vi "emi_ Loop multi error state monitor.vi"(5 "Loop ID in":u16, 9 "error in (no error)":errorcluster, 12 "Loc Sub ID":u16, 13 "Elevated priority":bool) -> (6 "Loop ID out":u16, 10 "error out":errorcluster)   [LabVIEW 2011]
doc: "Monitors severl error states based on sub id. Sends a message when any of them changes.\n\nDoes not remove teh errors"
uses:
  emi_Read System ID.vi
  Private/_emi_GFV System ID.vi
  <vilib>/Utility/error.llb/Clear Errors.vi
  S&E reporting/Private/_emi_S&E Q Generator.vi
panel:
  # "Always uses Sub ID 0."
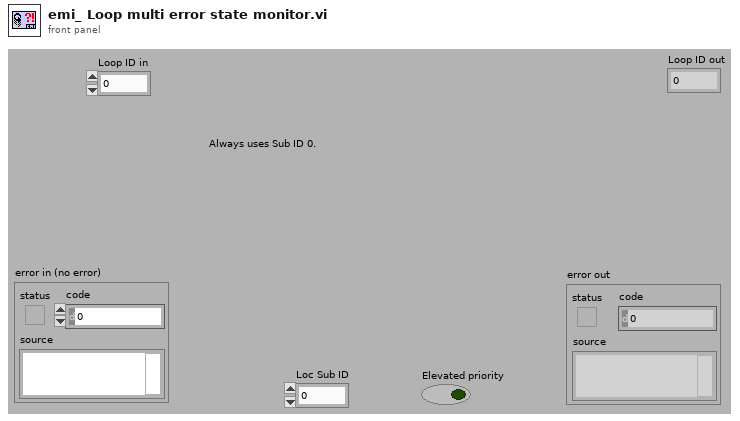
[diagram p1: front panel]
types:
  T1 = cluster{"error in (no error)":errorcluster, "Elevated priority":bool}
  T2 = cluster{"error in (no error)":errorcluster, "Elevated priority":bool}[]
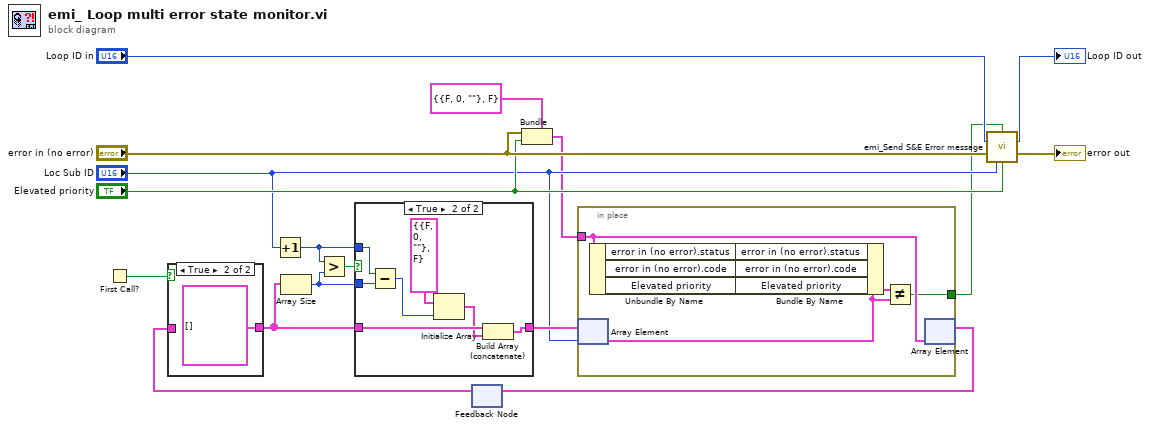
[diagram p0: block diagram]
diagram:
  n1 = First Call?() -> (First Call?: T/F=w8:bool)
  n2 = Increment(x="Loc Sub ID") -> (x+1=w9:u16)
  n3 = feedback #1() -> (w7:T2)  [unwired: 1 in]
  n4 = case shown="True" w8 {
    tunnel: [w18 T2 []] -> w6
    tunnel: w7 -> [w18 _]
    frame False {
    }
    frame True {
    }
  }
  n5 = Array Size(array=w6) -> (size(s)=w10:i32)
  n6 = Greater?(x=w9, y=w10) -> (0:w11:bool)
  n7 = case shown="True" w11 {
    tunnel: w10 -> [_ w26]
    tunnel: w9 -> [_ w27]
    tunnel: [w20 w22] -> w4
    tunnel: w6 -> [w20 w24]
    frame False {
    }
    frame True {
      n8 = Subtract(x=w27, y=w26) -> (x-y=w25:i32)
      n9 = Initialize Array(T1 {"error in (no error)"={"status"=FALSE, "code"=0, "source"=""}, "Elevated priority"=FALSE}, w25) -> (w23:T2)
      n10 = Build Array (concatenate)(w24, w23) -> (w22:T2)
    }
  }
  n11 = Bundle(cluster=T1 {"error in (no error)"={"status"=FALSE, "code"=0, "source"=""}, "Elevated priority"=FALSE}, "error in (no error)"="error in (no error)", "Elevated priority"="Elevated priority") -> (w2:T1)
  n12 = in-place {
    in-place-border: w2 -> [w29]
    in-place-border: [w28] -> w1
    n13 = in-place-array #2(w4, "Loc Sub ID") -> (w30:T1)
    n14 = Unbundle By Name(w29) -> ("error in (no error).status"=w34:bool, "error in (no error).code"=w33:i32, "Elevated priority"=w32:bool)
    n15 = Bundle By Name(cluster=w30, "error in (no error).status"=w34, "error in (no error).code"=w33, "Elevated priority"=w32) -> (w31:T1)
    n16 = Not Equal?(x=w31, y=w30) -> (x != y?=w28:bool)
    n17 = in-place-array #2(w29) -> (w5:T2)  [unwired: 1 out]
  }
  n18 = feedback-in #1(w5) -> ()
  n19 = call "emi_Send S&E Error message.vi"("Send(T)"=w1, "Loop ID in(No Loop)"="Loop ID in", "error in (no error)"="error in (no error)", "Var Index"="Loc Sub ID", "Elevated priority"="Elevated priority") -> ("Loop ID out"=→"Loop ID out":u16, "error out"=→"error out":errorcluster)  [unwired: 9 in]
